vi "Read Queued Processed Incoming Messages.vi"(6 "timeout in ms (-1)":i32=100, 8 "error in":errorcluster, 11 "j1939 queues":T1) -> (0 "error out":errorcluster, 2 "timed out?":bool, 3 "Frames":T2[](array[typedef]) {"payload" format="%x"; "timestamp" format="%<%.7X\n%x>T"; "type" items=["CAN Data"=0, "CAN Remote"=1, "CAN Bus Error"=2, "J1939 Data"=192, "Delay"=224, "Log Trigger"=225, "Start Trigger"=226]; "identifier" format="%x"})   [LabVIEW 2013, in "J1939.lvlib"]
uses:
  J1939.lvlib
  <vilib>/xnet/xnet.llb/XNET Frame CAN.ctl
  <vilib>/xnet/xnet.llb/XNET Frame Type CAN.ctl
  API Types/Setup Information Cluster.ctl
  API Types/CAN Outgoing Message Cluster.ctl
  API Types/Convert DTCs Cluster.ctl
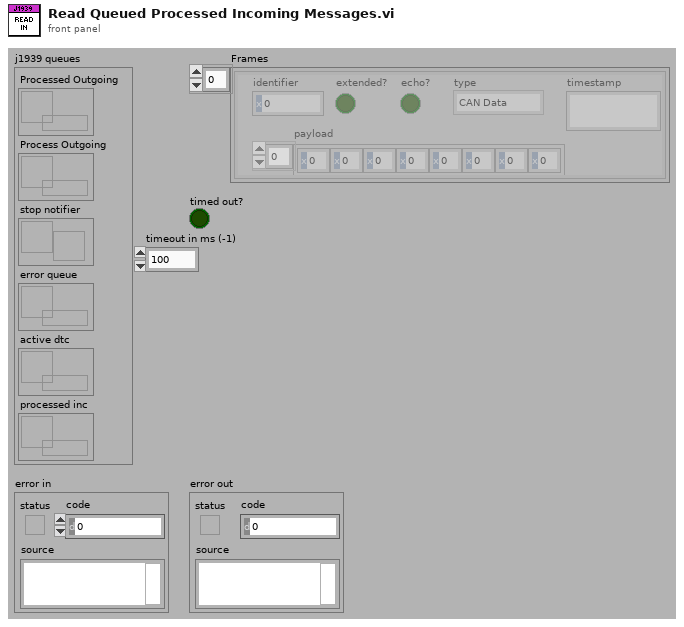
[diagram p1: front panel]
types:
  T1 = typedef "J1939.lvlib/Setup Information Cluster.ctl" = cluster{"Processed Outgoing":refnum<queue>, "Process Outgoing":refnum<queue>, "stop notifier":refnum<notifier>, "error queue":refnum<queue>, "active dtc":refnum<queue>, "processed inc":refnum<queue>}
  T2 = typedef "XNET Frame CAN.ctl" = cluster{"timestamp":timestamp, "payload":u8[], "identifier":u32, "type":T3, "extended?":bool, "echo?":bool}
  T3 = typedef "XNET Frame Type CAN.ctl" = u8
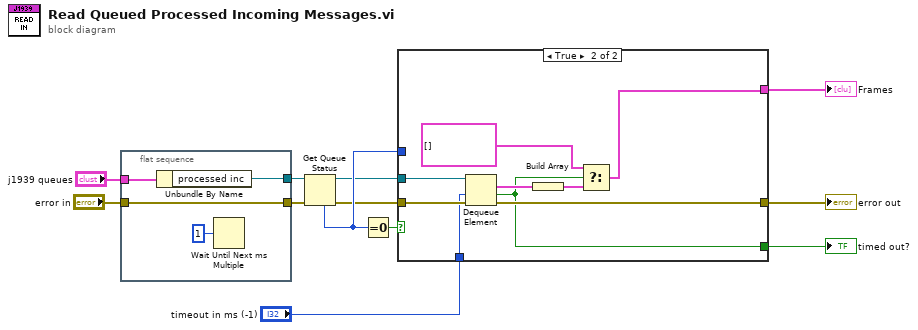
[diagram p0: block diagram]
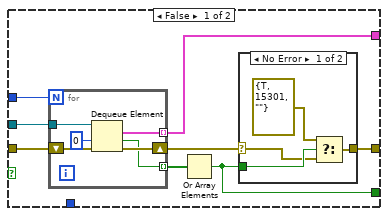
[diagram p2: hidden frame]
diagram:
  n1 = flat-sequence {
    tunnel: "j1939 queues" -> [w16]
    tunnel: [w14] -> w12
    tunnel: "error in" -> [w14]
    tunnel: [w13] -> w2
    frame #0 {
      n2 = Unbundle By Name(w16) -> ("processed inc"=w13:refnum<queue>)
      n3 = Wait Until Next ms Multiple(millisecond multiple=u32 1) -> ()  [unwired: 1 out]
    }
  }
  n4 = Get Queue Status(queue=w2, error in (no error)=w12) -> (queue out=w9:refnum<queue>, error out=w8:errorcluster, # elements in queue=w10:i32)  [unwired: 1 in, 5 out]
  n5 = Equal To 0?(x=w10) -> (x = 0?=w7:bool)
  n6 = case shown="True" w7 {
    tunnel: [w18 w43] -> w5
    tunnel: w9 -> [w24 w37]
    tunnel: w8 -> [w22 w44]
    tunnel: [w23 w38] -> w6
    tunnel: w10 -> [w21 _]
    tunnel: [w19 w39] -> w4
    tunnel: "timeout in ms (-1)" -> [_ w36]
    frame False {
      n7 = for {
        N: w21 -> [_]
        tunnel: w24 -> [w30]
        tunnel: [w34] -> w23 mode=indexing
        shift-right: [w35] -> w17
        shift-left: w22 -> [w33]
        tunnel: [w32] -> w20 mode=indexing
        n8 = Dequeue Element(queue=w30, timeout in ms (-1)=0, error in (no error)=w33) -> (element=w34:T2, timed out?=w32:bool, error out=w35:errorcluster)  [unwired: 1 out]
      }
      n9 = Or Array Elements(Boolean array=w20) -> (logical OR=w19:bool)
      n10 = case shown="No Error" w17 {
        selector: w17 -> [w25 w29]
        tunnel: w19 -> [w28 _]
        tunnel: [w27 w29] -> w18
        frame No Error {
          n11 = Select(t=errorcluster {"status"=TRUE, "code"=15301, "source"=""}, s=w28, f=w25) -> (s? t:f=w27:errorcluster)
        }
        frame Error {
        }
      }
    }
    frame True {
      n12 = Dequeue Element(queue=w37, timeout in ms (-1)=w36, error in (no error)=w44) -> (element=w42:T2, timed out?=w39:bool, error out=w43:errorcluster)  [unwired: 1 out]
      n13 = Build Array(w42) -> (w41:T2[])
      n14 = Select(t=T2[] [], s=w39, f=w41) -> (s? t:f=w38:T2[])
    }
  }
  "Frames" <- w6
  "error out" <- w5
  "timed out?" <- w4
